vi "clear Session Data.vi"(0 "OBJ - Measurement Session in":refnum<class "System Log.lvclass">, 11 "error in":errorcluster) -> (4 "OBJ - Measurement Session out":refnum<class "System Log.lvclass">, 15 "error out":errorcluster)   [LabVIEW 2016, in "System Log.lvclass"]
doc: "OVERRIDE VI\nPlaceholder for decendant classes to clear session information and close references."
uses:
  System Log.lvclass
  System Log.lvclass/System Log.ctl
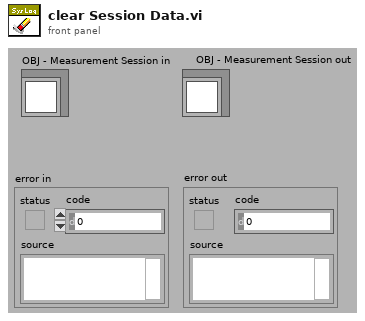
[diagram p1: front panel]
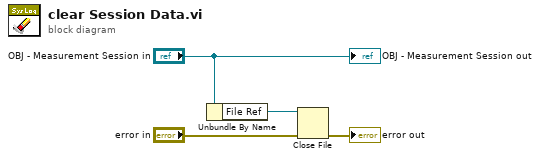
[diagram p0: block diagram]
diagram:
  n1 = Unbundle By Name("OBJ - Measurement Session in") -> ("File Ref"=w2:refnum<file>)
  n2 = Close File(refnum=w2, error in="error in") -> (error out=→"error out":errorcluster)  [unwired: 1 out]
  "OBJ - Measurement Session out" <- "OBJ - Measurement Session in"
